vi "FAA.vi"(0 "System no.":i32=1 min=1 step=1, 1 "Board":i32=1 min=1 max=5 step=1, 2 "Axis to scan":string, 4 "Range":dbl=0.1 format="%.4f", 5 "error in":errorcluster, 6 "Treshold level":dbl=0.1 format="%.3f", 8 "Decrease VEL\nfor scan?":bool=TRUE, 9 "Velocity":dbl=0.2 format="%.4f", 10 "Use #7 polling?":bool, 11 "Timeout (s)":dbl=300.0 min=1.0 max=4.0 step=1.0 format="%.2f", 12 "Stop refnum":refnum<vi>) -> (14 "Scan successful?":bool, 19 "error out":errorcluster)   [LabVIEW 2020]
doc: "Performs a fast angular line scan to maximum in specified axis, waits until scan is ready (using #7 polling if checked) and indicates whether scan was successful or not. Scan starts at (Current position - ½ Range) and stops at (Current position + ½ Range). \"Velocity\" is only valid if \"Decrease VEL for scan?\" is TRUE. If \"Decrease VEL for scan?\" is TRUE, velocity is decreased before and reset after the scan. \"Timeout\" is only valid if \"Use #7 polling\" is FALSE. If \"Refnum stop\" or \"Local stop\" is TRUE, VI resets velocity if it was decreased before, sends #24 and stops. \n\nC-887, F-206: Only for GCS syntax version = GCS 1.0 (check with CSV?.vi. If CSV?.vi is not supported, syntax version is GCS 1.0). For compatibility reasons, VI calls FLM automatically for GCS 2.0."
uses:
  Communication.llb/Syntax.ctl
  General command.llb/Controller names.ctl
  Communication.llb/Global1.vi
  General command.llb/Global2 (Array).vi
panel:
  out "Controller error":bool
  in  "Local stop":bool
  # "Performs a fast angular line scan to maximum in specified axis, waits until scan is ready (using #7 polling if checked) and \nindicates whether scan was successful or not. Scan starts at (Current position - ½ Range) and stops at (Current position \n+ ½ Range). \"Velocity\" is only valid if \"Decrease VEL for scan?\" Is TRUE. If \"Decrease VEL for scan?\" is TRUE, velocity is \ndecreased before and reset after the scan. \"Timeout\" is only valid if \"Use #7 polling\" is FALSE. If \"Stop refnum\" or \"Local \nstop\" is TRUE, VI resets velocity if it was decreased before, sends #24 and stops."
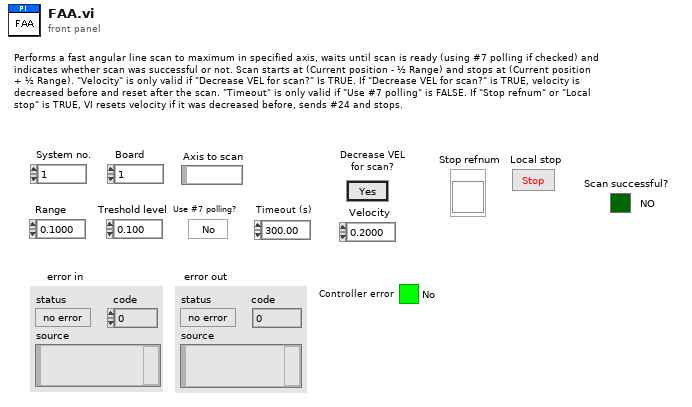
[diagram p1: front panel]
types:
  T1 = typedef "Syntax.ctl" = enum16{"GCS 1.0", "GCS 2.0", "GCS 3.0"}
  T2 = typedef "Controller names.ctl" = enum16{"None", "Analog", "C-702", "C-413", "C-414", "C-843", "C-843.PM", "C-844", "C-848", "C-865", "C-866", "C-867", "C-877", "C-880", "C-884", "C-885", "C-886", "C-887", "C-891", "E-135", "E-516", "E-517", "E-518", "E-709", "E-710", "E-712", "E-725", "E-727", "E-753", "E-754", "E-755", "E-761", "E-816", "E-861", "E-870", "E-871", "E-872", "E-873", "E-874", "F-206", "HydraPollux", "M-840", "M-850", "M-8X0", "Mercury", "Mercury_GCS", "PI_GCS2"}
  T3 = enum16{"Disable error check", "Force error check", "Use global settings"}
  T4 = cluster{"Conn. axes":string[], "Controller name":T2}[]
  T5 = cluster{"Conn. axes":string[], "Controller name":T2}
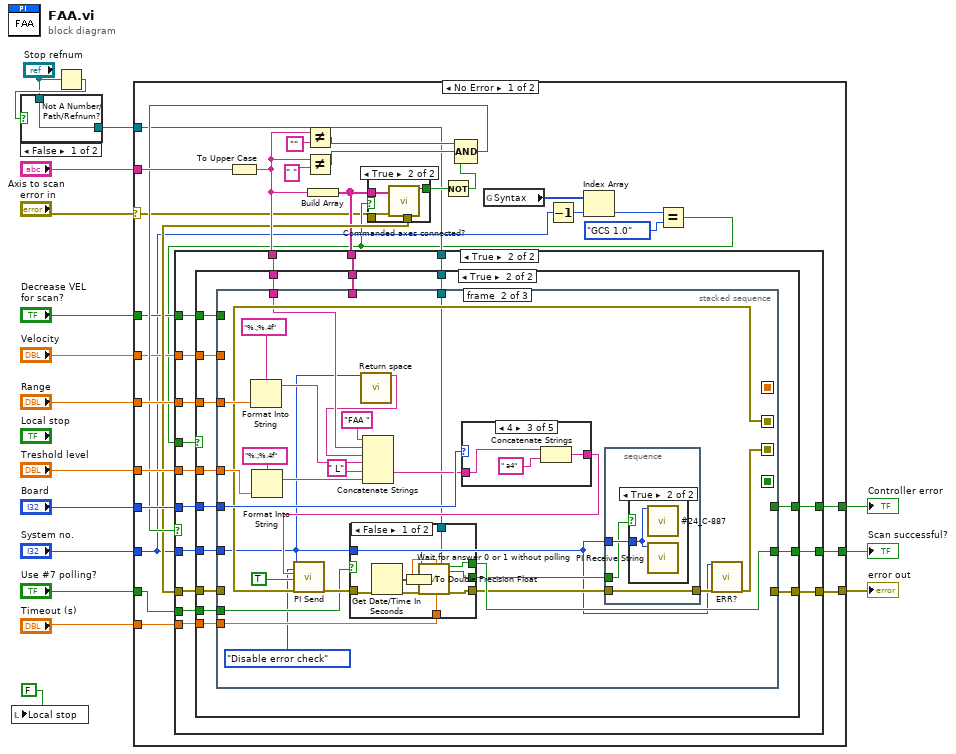
[diagram p0: block diagram]
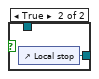
[diagram p2: hidden frame]
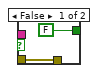
[diagram p3: hidden frame]
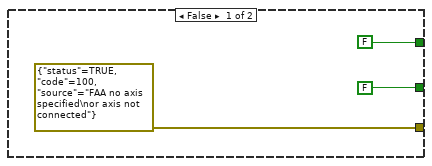
[diagram p4: hidden frame]
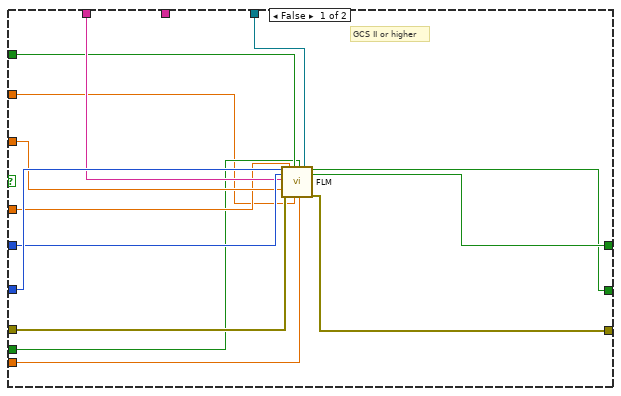
[diagram p5: hidden frame]
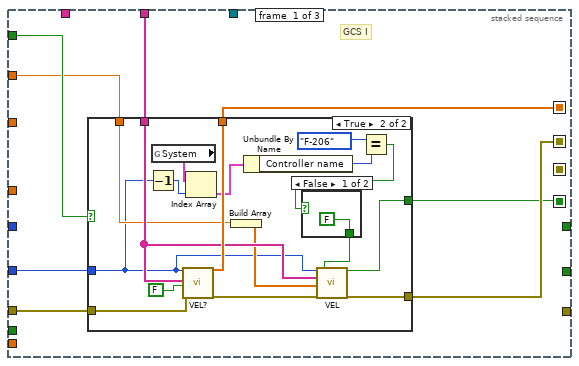
[diagram p6: hidden frame]
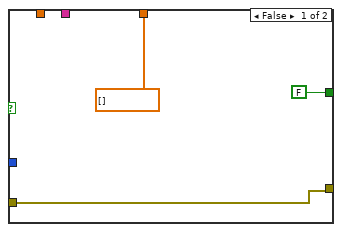
[diagram p7: hidden frame]
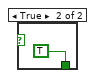
[diagram p8: hidden frame]
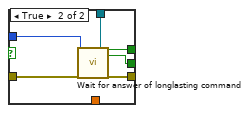
[diagram p9: hidden frame]
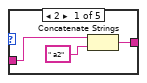
[diagram p11: hidden frame]
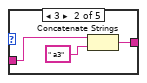
[diagram p12: hidden frame]
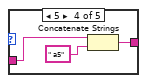
[diagram p13: hidden frame]
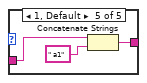
[diagram p14: hidden frame]
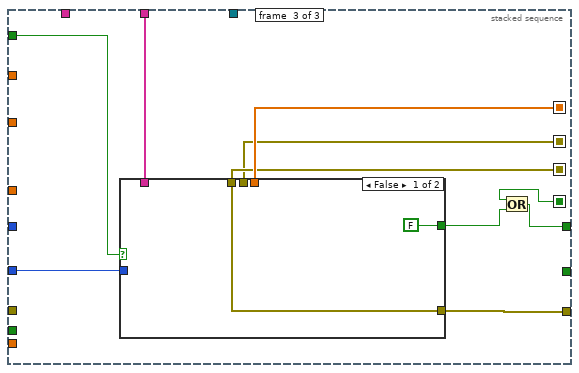
[diagram p15: hidden frame]
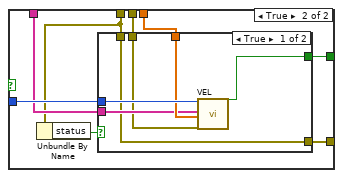
[diagram p16: hidden frame]
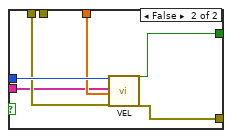
[diagram p17: hidden frame]
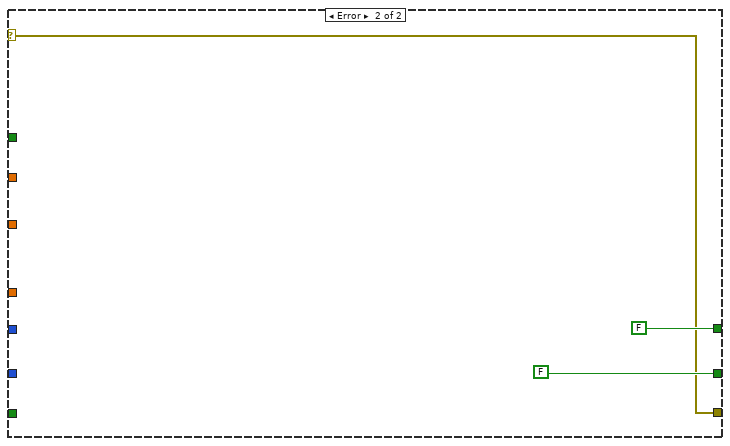
[diagram p18: hidden frame]
diagram:
  n1 = local write "Local stop"(FALSE ("Local stop")) -> ()
  n2 = Not A Number/Path/Refnum?(number/path/refnum="Stop refnum") -> (NaN/Path/Refnum?=w5:bool)
  n3 = case shown="False" w5 {
    tunnel: [w18 w19] -> w3
    tunnel: "Stop refnum" -> [w18 _]
    frame False {
    }
    frame True {
      n4 = control-ref of="Local stop"() -> (w19:refnum<vi>)
    }
  }
  n5 = case shown="No Error" "error in" {
    selector: "error in" -> [w21 w225]
    tunnel: "System no." -> [w23 _]
    tunnel: [w37 w225] -> w16
    tunnel: "Axis to scan" -> [w48 _]
    tunnel: [w36 FALSE] -> w14
    tunnel: "Board" -> [w43 _]
    tunnel: "Range" -> [w42 _]
    tunnel: "Treshold level" -> [w40 _]
    tunnel: "Decrease VEL\nfor scan?" -> [w32 _]
    tunnel: "Velocity" -> [w31 _]
    tunnel: [w30 FALSE ("Controller error")] -> w8
    tunnel: "Use #7 polling?" -> [w29 _]
    tunnel: "Timeout (s)" -> [w28 _]
    tunnel: w3 -> [w27 _]
    frame No Error {
      n6 = To Upper Case(1:w48) -> (0:w41:string)
      n7 = Not Equal?(x=w41, y="") -> (x != y?=w45:bool)
      n8 = Not Equal?(x=w41, y=" ") -> (x != y?=w44:bool)
      n9 = Build Array(w41) -> (w33:string[])
      n10 = global read "Global1.vi" "Syntax"() -> (w24:T1[])
      n11 = Decrement(x=w23) -> (x-1=w25:i32)
      n12 = Index Array(array=w24, index=w25) -> (element=w26:T1)
      n13 = Equal?(x=w26, y=Syntax."GCS 1.0") -> (x = y?=w22:bool)
      n14 = case shown="True" w22 {
        tunnel: w21 -> [w50 w54]
        tunnel: [w50 w53] -> w38
        tunnel: [FALSE ("Controller error") w52] -> w35
        tunnel: w33 -> [_ w51]
        frame False {
        }
        frame True {
          n15 = call "Commanded axes connected?.vi"("Commanded axes"=w51, "error in"=w54) -> ("Controller error"=w52:bool, "error out"=w53:errorcluster)  [unwired: 1 in, 15 out]
        }
      }
      n16 = Not(x=w35) -> (.not. x?=w34:bool)
      n17 = Compound Arithmetic op=AND(w45, w44, w34) -> (w39:bool)
      n18 = case shown="True" w39 {
        tunnel: w43 -> [_ w73]
        tunnel: w42 -> [_ w70]
        tunnel: w41 -> [_ w72]
        tunnel: w40 -> [_ w69]
        tunnel: w38 -> [_ w71]
        tunnel: w23 -> [_ w66]
        tunnel: [errorcluster {"status"=TRUE, "code"=100, "source"="FAA no axis specified\nor axis not connected"} ("error out") w67] -> w37
        tunnel: [FALSE w68] -> w36
        tunnel: w33 -> [_ w65]
        tunnel: w32 -> [_ w64]
        tunnel: w31 -> [_ w63]
        tunnel: [FALSE ("Controller error") w62] -> w30
        tunnel: w29 -> [_ w61]
        tunnel: w28 -> [_ w60]
        tunnel: w27 -> [_ w59]
        tunnel: w22 -> [_ w58]
        frame False {
        }
        frame True {
          n19 = case shown="True" w58 {
            tunnel: w73 -> [w86 w102]
            tunnel: w72 -> [w85 w101]
            tunnel: w71 -> [w83 w100]
            tunnel: w70 -> [w84 w99]
            tunnel: w69 -> [w82 w98]
            tunnel: [w74 w97] -> w68
            tunnel: [w76 w96] -> w67
            tunnel: w66 -> [w87 w95]
            tunnel: w65 -> [_ w94]
            tunnel: w64 -> [w81 w93]
            tunnel: w63 -> [w78 w92]
            tunnel: [w75 w91] -> w62
            tunnel: w61 -> [w80 w90]
            tunnel: w60 -> [w77 w89]
            tunnel: w59 -> [w79 w88]
            frame False {
              # "GCS II or higher"
              n20 = call "FLM.vi"("System no."=w87, "Board"=w86, "Axis to scan"=w85, "Range"=w84, "error in"=w83, "Treshold level"=w82, "Decrease VEL\nfor scan?"=w81, "Velocity"=w78, "Use #7 polling?"=w80, "Timeout (s)"=w77, "Stop refnum"=w79) -> ("Scan successful?"=w74:bool, "Controller error"=w75:bool, "error out"=w76:errorcluster)  [unwired: 2 in, 4 out]
            }
            frame True {
              n21 = stacked-sequence {
                seq-local: [w108 _ _] -> [_ _ w201]
                seq-local: [w106 _ _] -> [_ w143 w193]
                seq-local: [_ w142 _] -> [_ _ w199]
                seq-local: [w103 _ _] -> [_ _ w197]
                tunnel: w102 -> [_ w158 _]
                tunnel: w101 -> [_ w136 _]
                tunnel: w100 -> [w109 _ _]
                tunnel: w99 -> [_ w152 _]
                tunnel: w98 -> [_ w149 _]
                tunnel: [_ w148 _] -> w97
                tunnel: [_ _ w200] -> w96
                tunnel: w95 -> [w107 w135 w202]
                tunnel: w94 -> [w110 _ w198]
                tunnel: w93 -> [w105 _ w194]
                tunnel: w92 -> [w104 _ _]
                tunnel: [_ _ w195] -> w91
                tunnel: w90 -> [_ w141 _]
                tunnel: w89 -> [_ w140 _]
                tunnel: w88 -> [_ w139 _]
                frame #0 {
                  # "GCS I"
                  n22 = case shown="True" w105 {
                    tunnel: w110 -> [_ w125]
                    tunnel: w109 -> [w113 w129]
                    tunnel: [dbl[] [] ("Velocity") w128] -> w108
                    tunnel: w107 -> [_ w120]
                    tunnel: [w113 w126] -> w106
                    tunnel: w104 -> [_ w124]
                    tunnel: [FALSE ("Controller error") w122] -> w103
                    frame False {
                    }
                    frame True {
                      n23 = Decrement(x=w120) -> (x-1=w119:i32)
                      n24 = global read "Global2 (Array).vi" "System"() -> (w121:T4)
                      n25 = call "VEL?.vi"("System no."=w120, "Axes to query"=w125, "All axes?"=FALSE, "error in"=w129) -> ("Velocity"=w128:dbl[], "error out"=w127:errorcluster)  [unwired: 1 in, 13 out]
                      n26 = Index Array(array=w121, index=w119) -> (element=w118:T5)
                      n27 = Build Array(w124) -> (w123:dbl[])
                      n28 = Unbundle By Name(w118) -> ("Controller name"=w117:T2)
                      n29 = Equal?(x=Controller_names."F-206" ("Controller name"), y=w117) -> (x = y?=w115:bool)
                      n30 = case shown="False" w115 {
                        tunnel: [FALSE ("Without axis ID?") TRUE ("Without axis ID?")] -> w114
                        frame False {
                        }
                        frame True {
                        }
                      }
                      n31 = call "VEL.vi"("System no."=w120, "Axes to set"=w125, "Velocity values"=w123, "error in"=w127, "Without axis ID?"=w114) -> ("Controller error"=w122:bool, "error out"=w126:errorcluster)  [unwired: 1 in, 12 out]
                    }
                  }
                }
                frame #1 {
                  n32 = Format Into String(format string="%.;%.4f" ("Format String"), w152) -> (resulting string=w151:string)  [unwired: 2 in, 1 out]
                  n33 = Format Into String(format string="%.;%.4f" ("Format String"), w149) -> (resulting string=w144:string)  [unwired: 2 in, 1 out]
                  n34 = call "Return space.vi"("System no."=w135) -> ("String out"=w134:string)  [unwired: 1 in, 17 out]
                  n35 = Concatenate Strings("FAA ", w136, w134, w151, " L", w144) -> (w157:string)
                  n36 = case shown="4" w158 {
                    tunnel: w157 -> [w180 w183 w186 w189 w192]
                    tunnel: [w178 w181 w184 w187 w190] -> w156
                    frame 2 {
                      n37 = Concatenate Strings(w180, " a2" ("Substring")) -> (w178:string)
                    }
                    frame 3 {
                      n38 = Concatenate Strings(w183, " a3" ("Substring")) -> (w181:string)
                    }
                    frame 4 {
                      n39 = Concatenate Strings(w186, " a4" ("Substring")) -> (w184:string)
                    }
                    frame 5 {
                      n40 = Concatenate Strings(w189, " a5" ("Substring")) -> (w187:string)
                    }
                    frame 1, Default {
                      n41 = Concatenate Strings(w192, " a1" ("Substring")) -> (w190:string)
                    }
                  }
                  n42 = call "PI Send.vi"("System no."=w135, "Error check settings"=T3."Disable error check", "String to send"=w156, "Attach termination char.?"=TRUE ("Attach Linefeed?"), "error in"=w143) -> ("error out"=w154:errorcluster)  [unwired: 1 in, 13 out]
                  n43 = case shown="False" w141 {
                    tunnel: w154 -> [w164 w173]
                    tunnel: [w166 w172] -> w148
                    tunnel: [w165 w171] -> w147
                    tunnel: w135 -> [w162 w170]
                    tunnel: w140 -> [w163 _]
                    tunnel: w139 -> [w161 w169]
                    tunnel: [w160 w168] -> w138
                    frame False {
                      n44 = Get Date/Time In Seconds() -> (seconds since 1Jan1904=w159:timestamp)
                      n45 = To Double Precision Float(number=w159) -> (double precision float=w167:dbl)
                      n46 = call "Wait for answer 0 or 1 without polling.vi"("System no."=w162, "error in"=w164, "Start time"=w167, "Timeout (s)"=w163, "Stop refnum"=w161) -> ("Scan successful?"=w166:bool, "Stopped"=w160:bool, "error out"=w165:errorcluster)  [unwired: 12 out]
                    }
                    frame True {
                      n47 = call "Wait for answer of longlasting command.vi"("System no."=w170, "error in"=w173, "Stop refnum"=w169) -> ("Answer"=w172:bool, "Stopped"=w168:bool, "error out"=w171:errorcluster)  [unwired: 14 out]
                    }
                  }
                  n48 = stacked-sequence {
                    tunnel: w135 -> [w176]
                    tunnel: [w175] -> w146
                    tunnel: w147 -> [w175]
                    tunnel: w138 -> [w174]
                    frame #0 {
                      n49 = case shown="True" w174 {
                        tunnel: w176 -> [_ w177]
                        frame False {
                        }
                        frame True {
                          n50 = call "#24_C-887.vi"("System no."=w177) -> ()  [unwired: 1 in, 18 out]
                          n51 = call "PI Receive String.vi"("System no."=w177) -> ()  [unwired: 2 in, 17 out]
                        }
                      }
                    }
                  }
                  n52 = call "ERR?.vi"("System no."=w135, "error in"=w146) -> ("error out"=w142:errorcluster)  [unwired: 17 out]
                }
                frame #2 {
                  n53 = case shown="False" w194 {
                    tunnel: w202 -> [_ w212]
                    tunnel: w201 -> [_ w211]
                    tunnel: [w203 w210] -> w200
                    tunnel: w199 -> [w203 w205]
                    tunnel: w198 -> [_ w209]
                    tunnel: [FALSE ("Controller error") w208] -> w196
                    tunnel: w193 -> [_ w207]
                    frame False {
                    }
                    frame True {
                      n54 = Unbundle By Name(w205) -> ("status"=w206:bool)
                      n55 = case shown="True" w206 {
                        tunnel: w212 -> [w218 w224]
                        tunnel: w211 -> [w217 w223]
                        tunnel: [w213 w222] -> w210
                        tunnel: w205 -> [w213 w221]
                        tunnel: w209 -> [w216 w220]
                        tunnel: [w215 w219] -> w208
                        tunnel: w207 -> [w214 _]
                        frame True {
                          n56 = call "VEL.vi"("System no."=w218, "Axes to set"=w216, "Velocity values"=w217, "error in"=w214) -> ("Controller error"=w215:bool)  [unwired: 2 in, 13 out]
                        }
                        frame False {
                          n57 = call "VEL.vi"("System no."=w224, "Axes to set"=w220, "Velocity values"=w223, "error in"=w221) -> ("Controller error"=w219:bool, "error out"=w222:errorcluster)  [unwired: 2 in, 12 out]
                        }
                      }
                    }
                  }
                  n58 = Or(x=w197, y=w196) -> (x .or. y?=w195:bool)
                }
              }
            }
          }
        }
      }
    }
    frame Error {
    }
  }
  "error out" <- w16
  "Scan successful?" <- w14
  "Controller error" <- w8
